vi "Linear Envelope_Burst Study.vi"(1 "Signals":dbl[](array[numeric])) -> (0 "Filtered Signals":dbl[](array[numeric]))   [LabVIEW 2011]
uses:
  <vilib>/Analysis/NI_AALBase.lvlib
  <vilib>/Analysis/3filter.llb/Butterworth Filter (DBL).vi
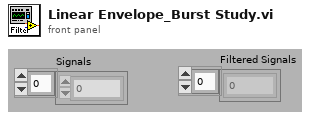
[diagram p1: front panel]
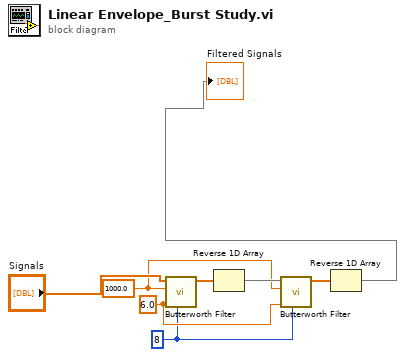
[diagram p0: block diagram]
diagram:
  w1 = 8 ("order")
  w3 = 1000.0 ("sampling freq: fs")
  w4 = 6.0 ("low cutoff freq: fl")
  n1 = call-poly <vilib>:"Butterworth Filter.vi"("order"=w1, "low cutoff freq: fl"=w4, "sampling freq: fs"=w3, "X"="Signals") -> ("Filtered X"=w6:dbl[])  [unwired: 4 in, 1 out]
  n2 = Reverse 1D Array(array=w6) -> (reversed array=w5:dbl[])
  n3 = call-poly <vilib>:"Butterworth Filter.vi"("order"=w1, "low cutoff freq: fl"=w4, "sampling freq: fs"=w3, "X"=w5) -> ("Filtered X"=w2:dbl[])  [unwired: 4 in, 1 out]
  n4 = Reverse 1D Array(array=w2) -> (reversed array=→"Filtered Signals":dbl[])
